vi "Create.vi"(10 "Size":cluster{"X":i32, "Y":i32}) -> (3 "Game Board out":refnum<class "Game Board.lvclass">)   [LabVIEW 2020, in "Game Board.lvclass"]
uses:
  Game Board.lvclass
  Game Board.lvclass/Game Board.ctl
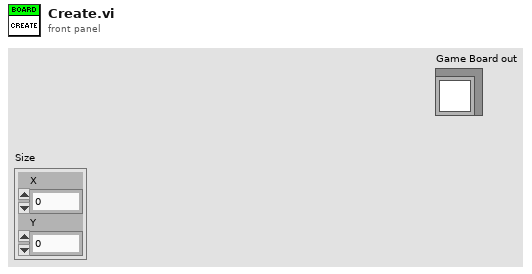
[diagram p1: front panel]
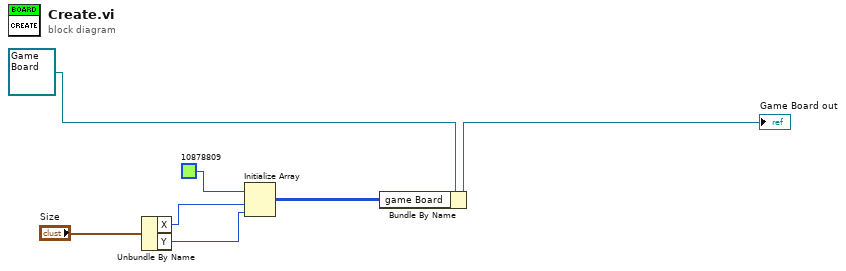
[diagram p0: block diagram]
diagram:
  n1 = Unbundle By Name("Size") -> ("X"=w3:i32, "Y"=w2:i32)
  n2 = Initialize Array(u32 10878809 ("Color Box"), w3, w2) -> (w1:u32[][])
  n3 = Bundle By Name(cluster=refnum<class "Game Board.lvclass"> refnum ("Game Board in"), "game Board"=w1) -> (→"Game Board out":refnum<class "Game Board.lvclass">)
